vi "RSZVB Set Trace Unit.vi"(8 "error in (no error)":errorcluster {"code" format="%.0x"}, 9 "Format (Power)":i32(ring) items=["Power", "Voltage"], 10 "Channel (1)":i32=1, 11 "VISA session":refnum<visa-resource-name>) -> (0 "error out":errorcluster {"code" format="%.0x"}, 3 "dup VISA session":refnum<visa-resource-name>)   [LabVIEW 2011]
doc: "This VI selects the physical unit of the displayed trace.\n\nRemote-control command(s):\nCALCulate<Chn>:FORMat:WQUType POWer | VOLTage"
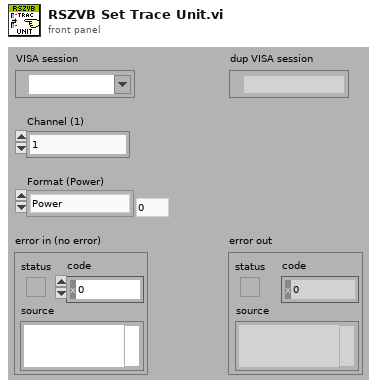
[diagram p1: front panel]
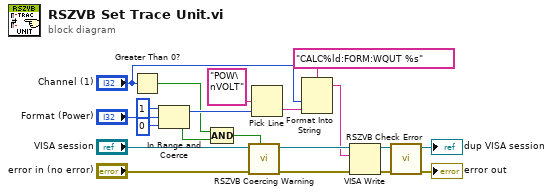
[diagram p0: block diagram]
diagram:
  n1 = Greater Than 0?(x="Channel (1)") -> (x > 0?=w11:bool)
  n2 = In Range and Coerce(upper limit=1, x="Format (Power)", lower limit=0) -> (coerced(x)=w18:i32, In Range?=w12:bool)
  n3 = Compound Arithmetic op=AND(w11, w12) -> (w10:bool)
  n4 = call "RSZVB Coercing Warning.vi"("In Range?"=w10, "error in (no error)"="error in (no error)", "VISA session"="VISA session") -> ("error out"=w16:errorcluster, "dup VISA session"=w17:refnum<visa-resource-name>)  [unwired: 7 in]
  n5 = Pick Line(multi-line string="POW\nVOLT", line index=w18) -> (output string=w13:string)  [unwired: 1 in]
  n6 = Format Into String(format string="CALC%ld:FORM:WQUT %s", "Channel (1)", w13) -> (resulting string=w9:string)  [unwired: 2 in, 1 out]
  n7 = VISA Write(VISA resource name=w17, write buffer=w9, error in (no error)=w16) -> (VISA resource name out=w14:refnum<visa-resource-name>, error out=w15:errorcluster)  [unwired: 1 out]
  n8 = call "RSZVB Check Error.vi"("error in (no error)"=w15, "VISA session"=w14) -> ("error out"=→"error out":errorcluster, "dup VISA session"=→"dup VISA session":refnum<visa-resource-name>)  [unwired: 8 in]
